vi "Drive Straight Pigeon Direct.vi"(4 "D Gain":dbl=5e-05 format="%#_13g", 6 "P Gain":dbl=0.0725 format="%#_13g", 7 "Max Corrective Throttle":dbl, 9 "Target angle":dbl format="%#_13g", 10 "Throttle":dbl format="%#_13g", 11 "Get All":T1 {"Calibration"."CurrentMode" items=["BootTareGryoAccel"=0, "Temperature"=1, "Magnetometer12Pt"=2, "Magnetometer360"=3, "Accelerometer"=5]}) -> (2 "Left Motor Value":dbl, 3 "Right Motor Value":dbl)   [LabVIEW 2016]
uses:
  <vilib>/Rock Robotics/WPI/ThirdParty/Sensors/Pigeon IMU/CTRE_PigeonIMU_GlobalStatus.ctl
  <vilib>/Rock Robotics/WPI/ThirdParty/Sensors/Pigeon IMU/CTRE_PigeonIMU_PigeonState.ctl
  <vilib>/Rock Robotics/WPI/ThirdParty/Sensors/Pigeon IMU/CTRE_PigeonIMU_CalibrationMode.ctl
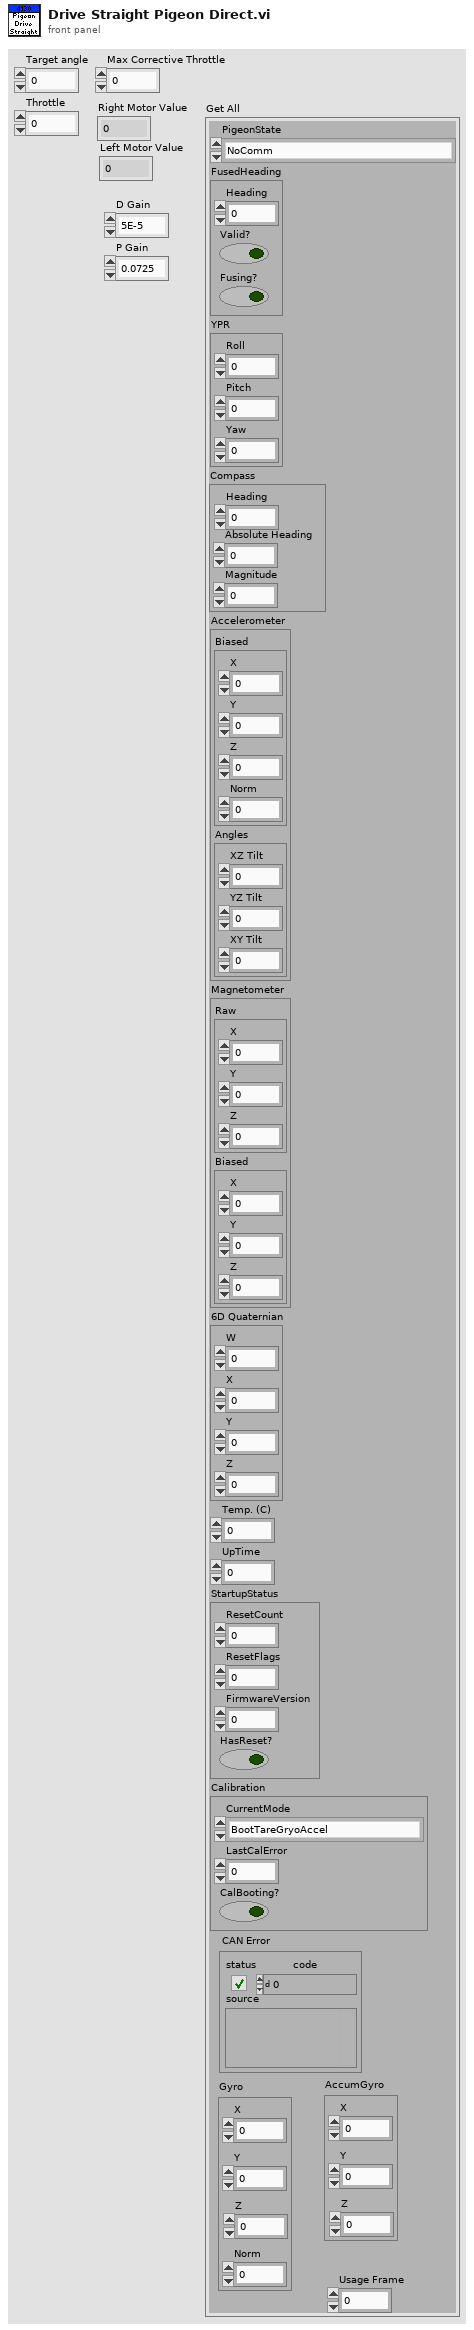
[diagram p1: front panel]
types:
  T1 = typedef "CTRE_PigeonIMU_GlobalStatus.ctl" = cluster{"PigeonState":T2, "FusedHeading":cluster{"Heading":dbl, "Valid?":bool, "Fusing?":bool}, "YPR":cluster{"Yaw":dbl, "Pitch":dbl, "Roll":dbl}, "Compass":cluster{"Heading":dbl, "Magnitude":dbl, "Absolute Heading":dbl}, "Accelerometer":cluster{"Biased":cluster{"X":i16, "Y":i16, "Z":i16, "Norm":i16}, "Angles":cluster{"XZ Tilt":dbl, "YZ Tilt":dbl, "XY Tilt":dbl}}, "Magnetometer":cluster{"Raw":cluster{"X":i16, "Y":i16, "Z":i16}, "Biased":cluster{"X":i16, "Y":i16, "Z":i16}}, "Gyro":cluster{"X":dbl, "Y":dbl, "Z":dbl, "Norm":dbl}, "6D Quaternian":cluster{"W":dbl, "X":dbl, "Y":dbl, "Z":dbl}, "Temp. (C)":dbl, "UpTime":u32, "StartupStatus":cluster{"ResetCount":i32, "ResetFlags":i32, "FirmwareVersion":i32, "HasReset?":bool}, "Calibration":cluster{"CurrentMode":T3, "LastCalError":i32, "CalBooting?":bool}, "CAN Error":errorcluster, "AccumGyro":cluster{"X":dbl, "Y":dbl, "Z":dbl}, "Usage Frame":u32}
  T2 = typedef "CTRE_PigeonIMU_PigeonState.ctl" = enum16{"NoComm", "Initializing", "Ready", "UserCalibration"}
  T3 = typedef "CTRE_PigeonIMU_CalibrationMode.ctl" = u16
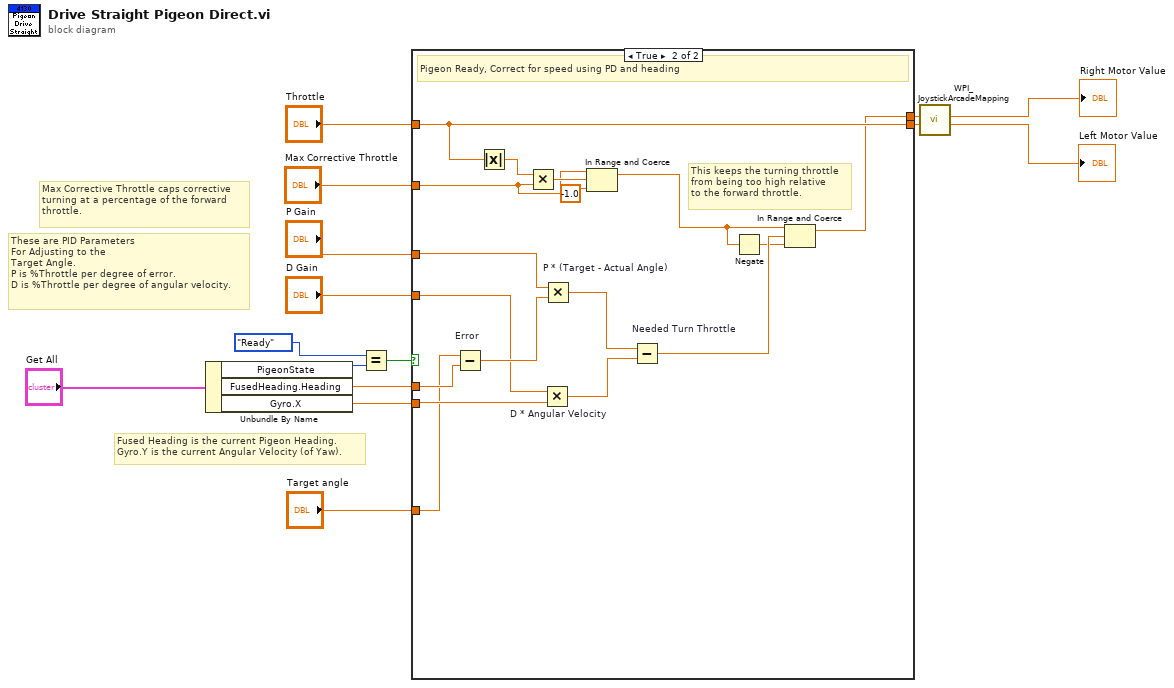
[diagram p0: block diagram]
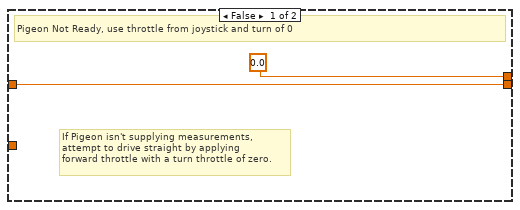
[diagram p2: hidden frame]
diagram:
  # "Fused Heading is the current Pigeon Heading.\nGyro.Y is the current Angular Velocity (of Yaw)."
  # "Max Corrective Throttle caps corrective\nturning at a percentage of the forward\nthrottle."
  # "These are PID Parameters\nFor Adjusting to the\nTarget Angle.\nP is %Throttle per degree of error.\nD is %Throttle per degree of angular velocity."
  n1 = Unbundle By Name("Get All") -> ("PigeonState"=w8:T2, "FusedHeading.Heading"=w7:dbl, "Gyro.X"=w6:dbl)
  n2 = Equal?(x=CTRE_PigeonIMU_PigeonState."Ready" ("PigeonState"), y=w8) -> (x = y?=w10:bool)
  n3 = case shown="True" w10 {
    tunnel: "Throttle" -> [w17 w26]
    tunnel: [w17 w26] -> w4
    tunnel: [0.0 ("upper limit") w20] -> w5
    tunnel: w7 -> [_ w34]
    tunnel: "Target angle" -> [_ w19]
    tunnel: w6 -> [_ w31]
    tunnel: "P Gain" -> [_ w32]
    tunnel: "D Gain" -> [_ w30]
    tunnel: "Max Corrective Throttle" -> [_ w18]
    frame False {
      # "If Pigeon isn't supplying measurements,\nattempt to drive straight by applying\nforward throttle with a turn throttle of zero."
      # "Pigeon Not Ready, use throttle from joystick and turn of 0"
    }
    frame True {
      # "This keeps the turning throttle\nfrom being too high relative\nto the forward throttle."
      # "Pigeon Ready, Correct for speed using PD and heading"
      n4 = Subtract "Error"(x=w19, y=w34) -> (x-y=w33:dbl)
      n5 = Absolute Value(x=w26) -> (abs(x)=w27:dbl)
      n6 = Multiply ("P * (Target - Actual Angle)")(x=w27, y=w18) -> (x*y=w24:dbl)
      n7 = Multiply "D * Angular Velocity"(x=w30, y=w31) -> (x*y=w28:dbl)
      n8 = Multiply "P * (Target - Actual Angle)"(x=w32, y=w33) -> (x*y=w29:dbl)
      n9 = In Range and Coerce(upper limit=w18, x=w24, lower limit=-1.0) -> (coerced(x)=w22:dbl)  [unwired: 1 out]
      n10 = Subtract "Needed Turn Throttle"(x=w29, y=w28) -> (x-y=w23:dbl)
      n11 = Negate(x=w22) -> (-x=w21:dbl)
      n12 = In Range and Coerce(upper limit=w22, x=w23, lower limit=w21) -> (coerced(x)=w20:dbl)  [unwired: 1 out]
    }
  }
  n13 = call <vilib>:"WPI_JoystickArcadeMapping.vi"("Y axis value"=w4, "X axis value"=w5) -> ("Right Motor Value"=→"Left Motor Value":dbl, "Left Motor Value"=→"Right Motor Value":dbl)  [unwired: 8 in]
